vi "CLD 9 Step Sequencer FGV Timer Solution.vi"() -> ()   [LabVIEW 2019]
doc: "CLD 9 Exercise"
uses:
  CLD 9 States .ctl
  CLD3 FGV Mode.ctl
panel:
  out "Current Step Time":dbl
  out "Elapsed Time (s)":string
  out "Step 3":bool
  out "Step 2":bool
  out "Step 1":bool
  out "Time Has Elapsed":bool
  in  "Auto Reset":bool=TRUE
  in  "Reset Button":bool
  in  "Stop VI":bool
  out "error out":errorcluster
  in  "error in (no error)":errorcluster
  in  "Time Target (s)":dbl
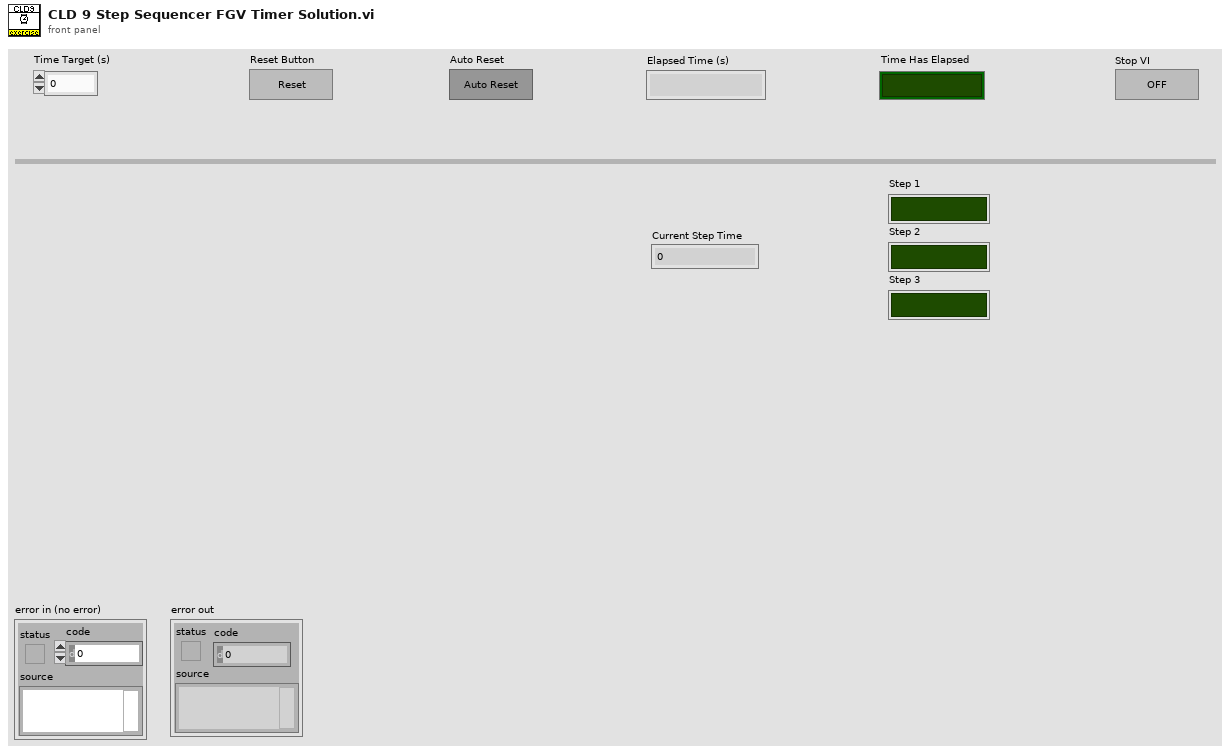
[diagram p1: front panel]
types:
  T1 = typedef "CLD 9 States .ctl" = enum16{"Start Step 1", "Step 1", "Start Step 2", "Step 2", "Start Step 3", "Step 3", "Check Auto Reset"}
  T2 = typedef "CLD3 FGV Mode.ctl" = enum16{"Start Timer", "Read Time", "Pause", "Resume", "Update Time Target (s)"}
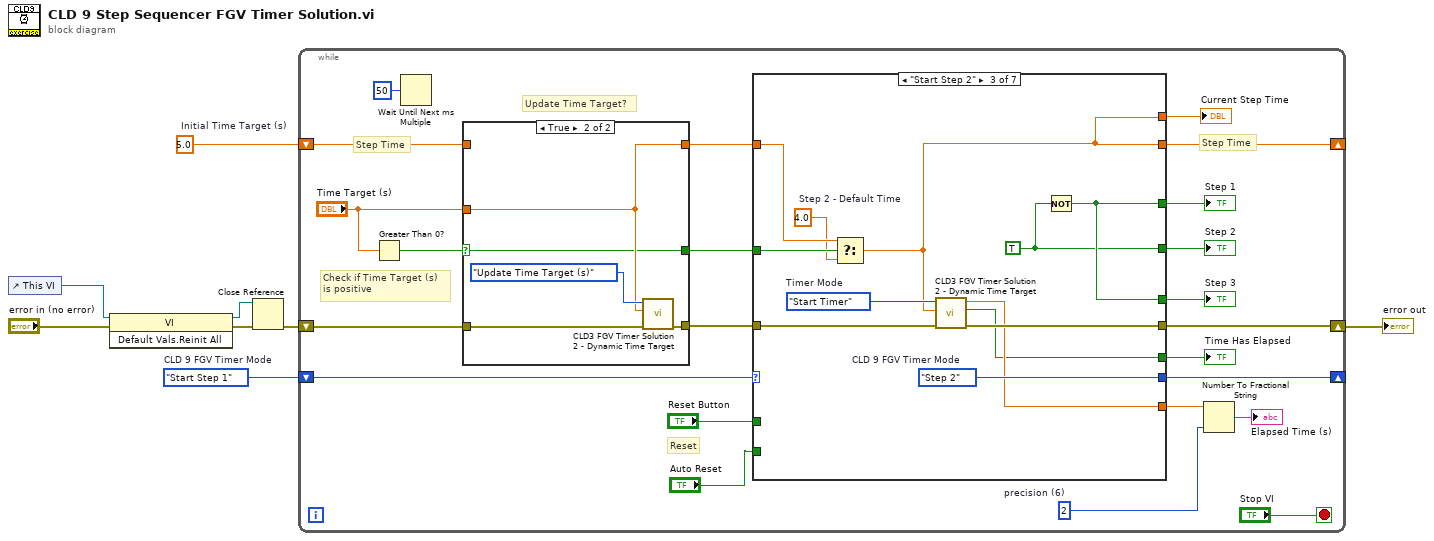
[diagram p0: block diagram]
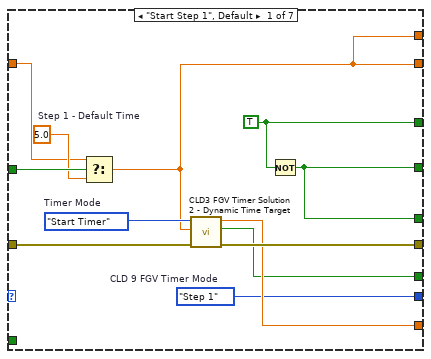
[diagram p3: hidden frame]
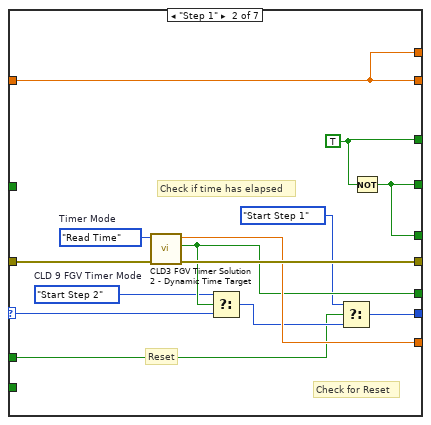
[diagram p4: hidden frame]
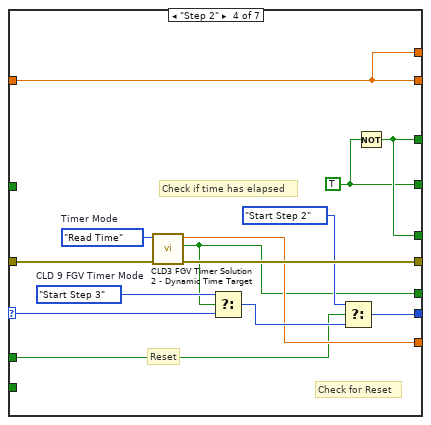
[diagram p5: hidden frame]
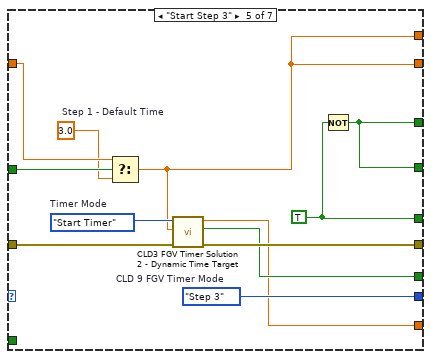
[diagram p6: hidden frame]
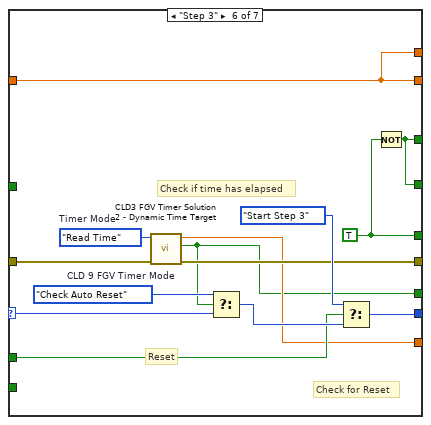
[diagram p7: hidden frame]
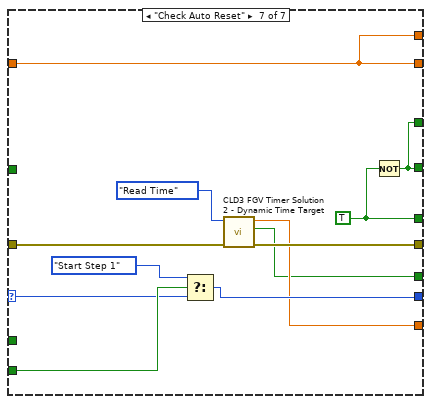
[diagram p8: hidden frame]
diagram:
  w1 = CLD_9_States_."Start Step 1"  # CLD 9 FGV Timer Mode
  w6 = 5.0  # Initial Time Target (s)
  n1 = control-ref of="This VI"() -> (w4:refnum<vi>)
  n2 = invoke class="VI" method="Default Vals.Reinit All"(reference=w4, error in="error in (no error)") -> (reference out=w2:refnum<vi>, error out=w5:errorcluster)  [unwired: 1 in, 1 out]
  n3 = Close Reference(reference=w2, error in (no error)=w5) -> (error out=w3:errorcluster)
  n4 = while {
    shift-right: [w22] -> w7
    shift-left: w3 -> [w30]
    shift-right: [w26] -> _
    shift-left: w6 -> [w28]
    shift-right: [w14] -> _
    shift-left: w1 -> [w25]
    stop <- "Stop VI" stop-if-true
    w16 = i16 2  # precision (6)
    # "Reset"
    # "Step Time"
    # "Step Time"
    # "Check if Time Target (s)\nis positive"
    # "Update Time Target?"
    n5 = Greater Than 0?(x="Time Target (s)") -> (x > 0?=w29:bool)
    n6 = Wait Until Next ms Multiple(millisecond multiple=u32 50) -> ()  [unwired: 1 out]
    n7 = case shown="True" w29 {
      selector: w29 -> [w32 w35]
      tunnel: w30 -> [w33 w39]
      tunnel: w28 -> [w34 _]
      tunnel: [w34 w36] -> w27
      tunnel: "Time Target (s)" -> [_ w36]
      tunnel: [w33 w38] -> w23
      tunnel: [w32 w35] -> w9
      frame False {
      }
      frame True {
        n8 = call "CLD3 FGV Timer Solution 2 - Dynamic Time Target.vi"("Error In"=w39, "Time Target (s)"=w36, "Timer Mode"=CLD3_FGV_Mode."Update Time Target (s)") -> ("Error Out"=w38:errorcluster)  [unwired: 6 in, 2 out]
      }
    }
    n9 = case shown="\"Start Step 2\"" w25 {
      selector: w25 -> [_ w58 _ w78 _ w111 w125]
      tunnel: w27 -> [w41 w52 w68 w80 w93 w103 w118]
      tunnel: [w40 w52 w66 w80 w91 w103 w118] -> w26
      tunnel: w23 -> [w50 w65 w76 w90 w101 w110 w122]
      tunnel: [w49 w64 w75 w90 w100 w109 w121] -> w22
      tunnel: [w45 w59 w72 w83 w98 w106 w119] -> w21
      tunnel: [w48 w61 w71 w82 w96 w104 w128] -> w20
      tunnel: [w47 w60 w70 w81 w96 w104 w128] -> w19
      tunnel: [w47 w60 w71 w82 w95 w105 w127] -> w18
      tunnel: [w46 w62 w73 w85 w97 w107 w120] -> w15
      tunnel: [w44 w55 w74 w84 w99 w108 w124] -> w14
      tunnel: "Reset Button" -> [_ w54 _ w79 _ w112 _]
      tunnel: [w40 w52 w66 w80 w91 w103 w118] -> w12
      tunnel: "Auto Reset" -> [_ _ _ _ _ _ w126]
      tunnel: w9 -> [w43 _ w69 _ w94 _ _]
      frame "Start Step 1", Default {
        w44 = CLD_9_States_."Step 1"  # CLD 9 FGV Timer Mode
        w48 = TRUE
        w51 = CLD3_FGV_Mode."Start Timer"  # Timer Mode
        w42 = 5.0  # Step 1 - Default Time
        n10 = Select(t=w41, s=w43, f=w42) -> (s? t:f=w40:dbl)
        n11 = call "CLD3 FGV Timer Solution 2 - Dynamic Time Target.vi"("Error In"=w50, "Time Target (s)"=w40, "Timer Mode"=w51) -> ("Error Out"=w49:errorcluster, "Has Time Elapsed"=w45:bool, "Elapsed Time (s.ss)"=w46:dbl)  [unwired: 6 in]
        n12 = Not(x=w48) -> (.not. x?=w47:bool)
      }
      frame "Step 1" {
        w57 = CLD_9_States_."Start Step 2"  # CLD 9 FGV Timer Mode
        w61 = TRUE
        w63 = CLD3_FGV_Mode."Read Time"  # Timer Mode
        # "Check for Reset"
        # "Check if time has elapsed"
        # "Reset"
        n13 = call "CLD3 FGV Timer Solution 2 - Dynamic Time Target.vi"("Error In"=w65, "Timer Mode"=w63) -> ("Error Out"=w64:errorcluster, "Has Time Elapsed"=w59:bool, "Elapsed Time (s.ss)"=w62:dbl)  [unwired: 7 in]
        n14 = Select(t=w57, s=w59, f=w58) -> (s? t:f=w56:T1)
        n15 = Select(t=CLD_9_States_."Start Step 1", s=w54, f=w56) -> (s? t:f=w55:T1)
        n16 = Not(x=w61) -> (.not. x?=w60:bool)
      }
      frame "Start Step 2" {
        w74 = CLD_9_States_."Step 2"  # CLD 9 FGV Timer Mode
        w70 = TRUE
        w77 = CLD3_FGV_Mode."Start Timer"  # Timer Mode
        w67 = 4.0  # Step 2 - Default Time
        n17 = Select(t=w68, s=w69, f=w67) -> (s? t:f=w66:dbl)
        n18 = call "CLD3 FGV Timer Solution 2 - Dynamic Time Target.vi"("Error In"=w76, "Time Target (s)"=w66, "Timer Mode"=w77) -> ("Error Out"=w75:errorcluster, "Has Time Elapsed"=w72:bool, "Elapsed Time (s.ss)"=w73:dbl)  [unwired: 6 in]
        n19 = Not(x=w70) -> (.not. x?=w71:bool)
      }
      frame "Step 2" {
        w88 = CLD_9_States_."Start Step 3"  # CLD 9 FGV Timer Mode
        w81 = TRUE
        w89 = CLD3_FGV_Mode."Read Time"  # Timer Mode
        # "Check for Reset"
        # "Check if time has elapsed"
        # "Reset"
        n20 = call "CLD3 FGV Timer Solution 2 - Dynamic Time Target.vi"("Timer Mode"=w89) -> ("Has Time Elapsed"=w83:bool, "Elapsed Time (s.ss)"=w85:dbl)  [unwired: 8 in, 1 out]
        n21 = Select(t=w88, s=w83, f=w78) -> (s? t:f=w87:T1)
        n22 = Select(t=CLD_9_States_."Start Step 2", s=w79, f=w87) -> (s? t:f=w84:T1)
        n23 = Not(x=w81) -> (.not. x?=w82:bool)
      }
      frame "Start Step 3" {
        w99 = CLD_9_States_."Step 3"  # CLD 9 FGV Timer Mode
        w95 = TRUE
        w102 = CLD3_FGV_Mode."Start Timer"  # Timer Mode
        w92 = 3.0  # Step 1 - Default Time
        n24 = Select(t=w93, s=w94, f=w92) -> (s? t:f=w91:dbl)
        n25 = call "CLD3 FGV Timer Solution 2 - Dynamic Time Target.vi"("Error In"=w101, "Time Target (s)"=w91, "Timer Mode"=w102) -> ("Error Out"=w100:errorcluster, "Has Time Elapsed"=w98:bool, "Elapsed Time (s.ss)"=w97:dbl)  [unwired: 6 in]
        n26 = Not(x=w95) -> (.not. x?=w96:bool)
      }
      frame "Step 3" {
        w115 = CLD_9_States_."Check Auto Reset"  # CLD 9 FGV Timer Mode
        w105 = TRUE
        w116 = CLD3_FGV_Mode."Read Time"  # Timer Mode
        # "Check for Reset"
        # "Check if time has elapsed"
        # "Reset"
        n27 = call "CLD3 FGV Timer Solution 2 - Dynamic Time Target.vi"("Error In"=w110, "Timer Mode"=w116) -> ("Error Out"=w109:errorcluster, "Has Time Elapsed"=w106:bool, "Elapsed Time (s.ss)"=w107:dbl)  [unwired: 7 in]
        n28 = Select(t=w115, s=w106, f=w111) -> (s? t:f=w114:T1)
        n29 = Select(t=CLD_9_States_."Start Step 3", s=w112, f=w114) -> (s? t:f=w108:T1)
        n30 = Not(x=w105) -> (.not. x?=w104:bool)
      }
      frame "Check Auto Reset" {
        w127 = TRUE
        n31 = Select(t=CLD_9_States_."Start Step 1", s=w126, f=w125) -> (s? t:f=w124:T1)
        n32 = call "CLD3 FGV Timer Solution 2 - Dynamic Time Target.vi"("Error In"=w122, "Timer Mode"=CLD3_FGV_Mode."Read Time") -> ("Error Out"=w121:errorcluster, "Has Time Elapsed"=w119:bool, "Elapsed Time (s.ss)"=w120:dbl)  [unwired: 7 in]
        n33 = Not(x=w127) -> (.not. x?=w128:bool)
      }
    }
    "Step 1" <- w20
    "Step 2" <- w19
    "Step 3" <- w18
    "Current Step Time" <- w12
    "Time Has Elapsed" <- w21
    n34 = Number To Fractional String(number=w15, precision (6)=w16) -> (F-format string=→"Elapsed Time (s)":string)  [unwired: 2 in]
  }
  "error out" <- w7
